vi "UpdateTypedefCluster.vi"(8 "error in (no error)":errorcluster, 9 "Delete Existing Controls":bool=TRUE, 10 "Control Refnums To Insert":refnum<vi>[](array[refnum]), 11 "Typedef Cluster":refnum<vi>) -> (0 "error out":errorcluster, 3 "Typedef Cluster out":refnum<vi>)   [LabVIEW 2020]
uses:
  <vilib>/Utility/miscctls.llb/LVPointTypeDef.ctl
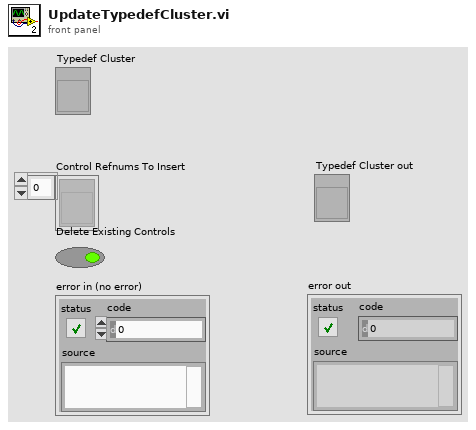
[diagram p1: front panel]
types:
  T1 = typedef "LVPointTypeDef.ctl" = cluster{"Horizontal":i16, "Vertical":i16}
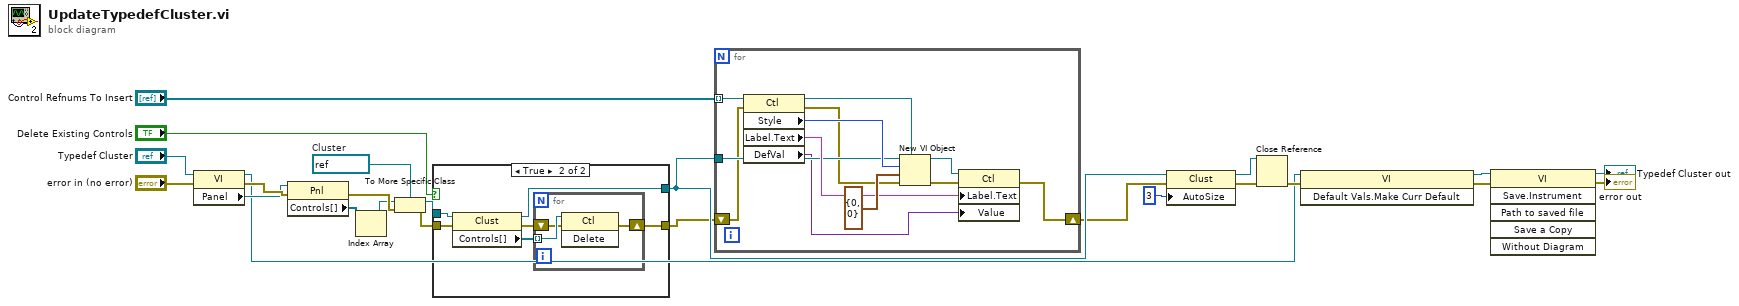
[diagram p0: block diagram]
diagram:
  w19 = refnum<vi> refnum  # Cluster
  n1 = property class="VI"(reference="Typedef Cluster", error in="error in (no error)") -> (reference out=w12:refnum<vi>, error out=w22:errorcluster, "Panel"=w16:refnum<vi>)
  n2 = property class="Pnl"(reference=w16, error in=w22) -> (error out=w23:errorcluster, "Controls[]"=w17:refnum<vi>[])  [unwired: 1 out]
  n3 = Index Array(array=w17) -> (element=w18:refnum<vi>)  [unwired: 1 in]
  n4 = To More Specific Class(target class=w19, reference=w18, error in=w23) -> (specific class reference=w20:refnum<vi>, error out=w24:errorcluster)
  n5 = case shown="True" "Delete Existing Controls" {
    tunnel: w24 -> [w25 w32]
    tunnel: [w26 w31] -> w21
    tunnel: w20 -> [w26 w30]
    tunnel: [w25 w29] -> w7
    frame False {
    }
    frame True {
      n6 = property class="Clust"(reference=w30, error in=w32) -> (reference out=w31:refnum<vi>, error out=w28:errorcluster, "Controls[]"=w27:refnum<vi>[])
      n7 = for {
        tunnel: w27 -> [w35] mode=indexing
        shift-right: [w33] -> w29
        shift-left: w28 -> [w34]
        n8 = invoke class="Ctl" method="Delete"(reference=w35, error in=w34) -> (error out=w33:errorcluster)  [unwired: 1 in, 2 out]
      }
    }
  }
  n9 = for {
    tunnel: w21 -> [w43]
    shift-right: [w41] -> w8
    shift-left: w7 -> [w39]
    tunnel: "Control Refnums To Insert" -> [w40] mode=indexing
    n10 = property class="Ctl"(reference=w40, error in=w39) -> (reference out=w36:refnum<vi>, error out=w38:errorcluster, "Style"=w47:u32, "Label.Text"=w44:string, "DefVal"=w37:variant)
    n11 = New VI Object(vi object class=w36, owner refnum=w43, style=w47, position/next to=T1 {"Horizontal"=0, "Vertical"=0} ("location"), 8:w38) -> (object refnum=w45:refnum<vi>, 0:w42:errorcluster)  [unwired: 3 in]
    n12 = property class="Ctl"(reference=w45, error in=w42, "Label.Text"=w44, "Value"=w37) -> (error out=w41:errorcluster)  [unwired: 1 out]
  }
  n13 = property class="Clust"(reference=w21, error in=w8, "AutoSize"=u32 3 ("Auto Sizing")) -> (reference out=w11:refnum<vi>, error out=w10:errorcluster)
  n14 = Close Reference(reference=w11, error in (no error)=w10) -> (error out=w14:errorcluster)
  n15 = invoke class="VI" method="Default Vals.Make Curr Default"(reference=w12, error in=w14) -> (reference out=w13:refnum<vi>, error out=w15:errorcluster)  [unwired: 1 in, 1 out]
  n16 = invoke class="VI" method="Save.Instrument"(reference=w13, error in=w15) -> (reference out=→"Typedef Cluster out":refnum<vi>, error out=→"error out":errorcluster)  [unwired: 4 in, 4 out]
